vi "PC_Pub_imgFile setRefnum.vi"(8 "error in (no error)":errorcluster, 10 "refnum":T1, 11 "imgFile in":refnum<class "PC_Pub_imgFile.lvclass">) -> (0 "error out":errorcluster, 3 "imgFile out":refnum<class "PC_Pub_imgFile.lvclass">)   [LabVIEW 2018, in "PC_Pub_imgFile.lvclass"]
uses:
  PC_Pub_imgFile.lvclass
  PC_Pub_imgFile.lvclass/PC_Pub_imgFile.ctl
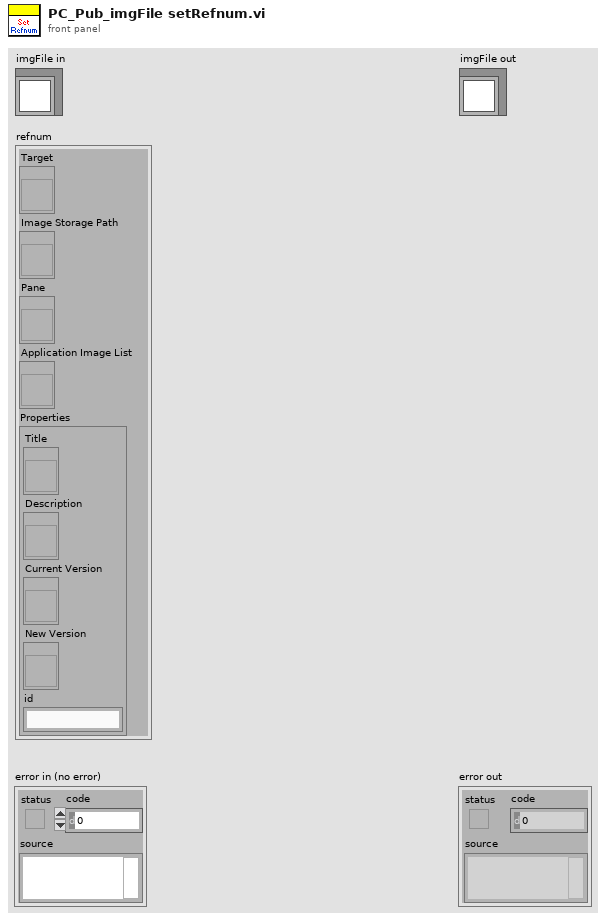
[diagram p1: front panel]
types:
  T1 = cluster{"Target":refnum<vi>, "Image Storage Path":refnum<vi>, "Pane":refnum<vi>, "Application Image List":refnum<vi>, "Properties":cluster{"Title":refnum<vi>, "Description":refnum<vi>, "Current Version":refnum<vi>, "New Version":refnum<vi>, "id":string}}
  T2 = cluster{"Title":refnum<vi>, "Description":refnum<vi>, "Current Version":refnum<vi>, "New Version":refnum<vi>, "id":string}
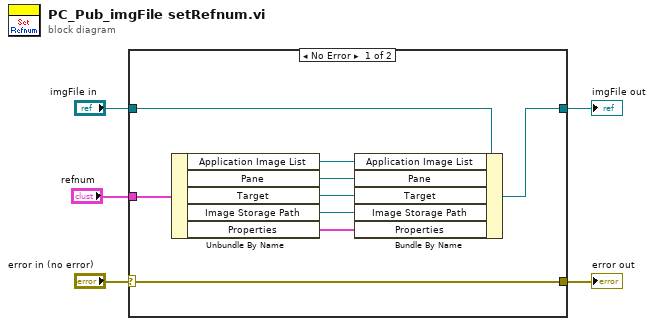
[diagram p0: block diagram]
diagram:
  n1 = case shown="No Error" "error in (no error)" {
    selector: "error in (no error)" -> [w14 w16]
    tunnel: [w14 w16] -> w4
    tunnel: [w8 w15] -> w2
    tunnel: "imgFile in" -> [w13 w15]
    tunnel: "refnum" -> [w12 _]
    frame No Error {
      n2 = Unbundle By Name(w12) -> ("Application Image List"=w6:refnum<vi>, "Pane"=w7:refnum<vi>, "Target"=w11:refnum<vi>, "Image Storage Path"=w10:refnum<vi>, "Properties"=w9:T2)
      n3 = Bundle By Name(cluster=w13, "Application Image List"=w6, "Pane"=w7, "Target"=w11, "Image Storage Path"=w10, "Properties"=w9) -> (w8:refnum<class "PC_Pub_imgFile.lvclass">)
    }
    frame Error {
    }
  }
  "error out" <- w4
  "imgFile out" <- w2
